vi "non-test.vi"() -> ()   [LabVIEW 2023]
uses:
  target/debug/liblabview_test_library.dylib
panel:
  out "return type":i32
  out "string":string
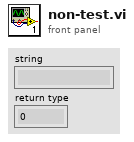
[diagram p1: front panel]
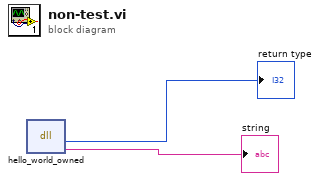
[diagram p0: block diagram]
diagram:
  n1 = dll-call lib="Volumes/NuFlo/work/src/Rust-LabVIEW-Interop/target/debug/liblabview_test_library.dylib" fn="hello_world_owned"() -> ("return type"=→"return type":i32, "string"=→"string":string)  [unwired: 4 in, 2 out]
